vi "Trigger B.vi"(6 "Slope":i32(ring) items=["Rising Edge", "Falling Edge"], 7 "Level":dbl, 8 "error in":errorcluster, 9 "Trigger Source":T1 items=["TTL0", "TTL1", "TTL2", "TTL3", "TTL4", "TTL5", "TTL6", "TTL7", "ECL0", "ECL1", "CH1 Trig", "CH2 Trig", "CH3 Trig", "CH4 Trig", "Ext", "Star", "Man", "Patt Trig"], 10 "State":i32(ring) items=["Enable", "Disable"], 11 "Instrument Handle In":i32) -> (0 "error out":errorcluster, 3 "Instrument Handle Out":i32)   [LabVIEW 8.6, in "ZTScopeM.lvlib"]
doc: "Configure the second edge trigger event qualifier."
uses:
  ZTScopeM.lvlib
  Trigger Source.ctl
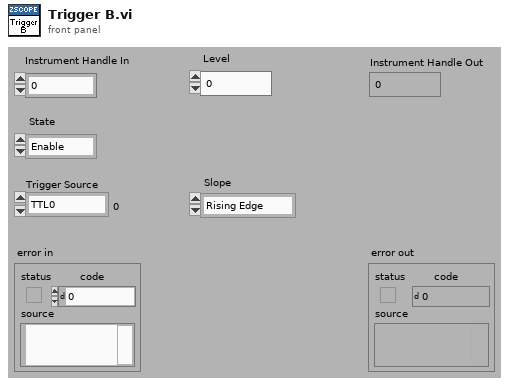
[diagram p1: front panel]
types:
  T1 = typedef "ZTScopeM.lvlib/Trigger Source.ctl" = i32
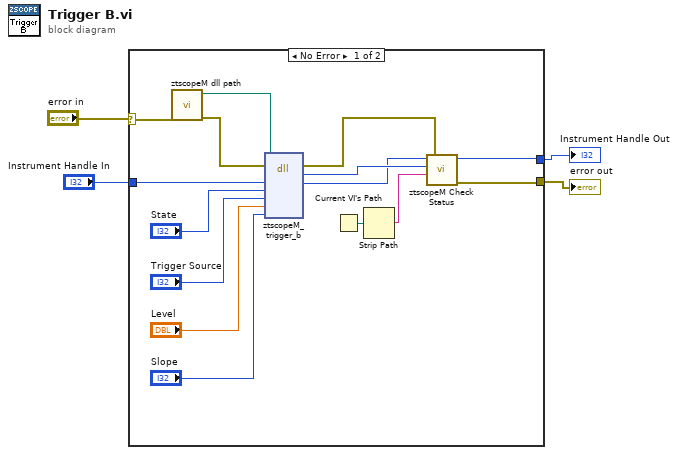
[diagram p0: block diagram]
diagram:
  n1 = case shown="No Error" "error in" {
    selector: "error in" -> [w8 w21]
    tunnel: [w9 w21] -> w1
    tunnel: "Instrument Handle In" -> [w19 w20]
    tunnel: [w10 w20] -> w2
    frame #0 {
      n2 = call "ztscopeM dll path.vi"("error in (no error)"=w8) -> ("error out"=w6:errorcluster, "<instrument>.dll path"=w7:path)  [unwired: 9 in]
      n3 = dll-call lib="C:/Program Files (x86)/National Instruments/LabVIEW 2013/instr.lib/ztscopem/ztscopeM.dll" fn="ztscopeM_trigger_b"(path in=w7, error in=w6, "instrumentHandle"=w19, "state"="State", "triggerSource"="Trigger Source", "level"="Level", "slope"="Slope") -> (error out=w5:errorcluster, w12:i32, "instrumentHandle"=w11:i32)  [unwired: 5 in, 1 out]
      n4 = Current VI's Path() -> (path=w14:path)
      n5 = Strip Path(path=w14) -> (name=w13:string)  [unwired: 1 out]
      n6 = call "ztscopeM Check Status.vi"("error in"=w5, "name of VI"=w13, "status (return code)"=w12, "instrument handle in"=w11) -> ("error out"=w9:errorcluster, "instrument handle out"=w10:i32)  [unwired: 2 in]
    }
    frame #1 {
    }
  }
  "Instrument Handle Out" <- w2
  "error out" <- w1
